vi "SequenceCtrl_HSImaging.vi"(0 "QueuesRef":T2, 1 "MotionStageRefs":refnum<queue>, 2 "AppsRef":refnum<queue>, 3 "subprog_Ref":refnum<vi>, 4 "TotalScan":i32, 5 "SecondaryVI_Ref":refnum<vi>, 7 "Params.":variant, 9 "Laser_Ctrl":bool, 10 "SecendaryParams":variant caption="SecendaryParams (Input)", 11 "error in":errorcluster, 12 "HighSpeed":dbl=5.0, 13 "LowSpeed":dbl=0.1, 14 "Single/MultiRec (T:M)":bool) -> (6 "Interupted":bool, 15 "error out":errorcluster)   [LabVIEW 2014]
uses:
  ControlDef/QueueRefs.ctl
  ControlDef/LaserCtrl_Method.ctl
  ControlDef/States-AToF.ctl
  <instrlib>/GenericDAQ/VI/GenericDAQ_Ctrl_Queue.ctl
  <instrlib>/GenericDAQ/VI/GenericDAQ_State.ctl
  <instrlib>/ESP300/Public/Data/ESP300_State.ctl
  <instrlib>/DG535/Command/DG535_States.ctl
  Hardware/BNC(QuantumComposers)/BNC_States.ctl
  Hardware/FemtoLaser(Legacy)/Laser_Status.ctl
  Hardware/DAQmx(Legacy)/DAQmx_Status.ctl
  ControlDef/Signal.ctl
  ProcessMethods/SignalAverager/ProcessStates.ctl
  Files/WriterState.ctl
  <instrlib>/GenericDAQ/VI/GenericDAQ_Signal.ctl
  Hardware/EPM2000(Legacy)/EPM2K_Status.ctl
  Apps_static/MeanderLoopState.ctl
  SequenceCtrl_State.ctl
  Apps_static/ScanParams_SingleLine.ctl
  <instrlib>/ESP300/Public/Data/ESP30x_Data.ctl
  <vilib>/Utility/error.llb/DialogType.ctl
  <instrlib>/GenericDAQ/VI/InstrParams.vi
  ControlDef/PauseMeander.vi
  <instrlib>/ESP300/ESP300.lvlib
  <instrlib>/DG535/SRS_DG535_Lib.lvlib
  <userlib>/Utility/ErrorLog_lib.lvlib
  <instrlib>/GenericDAQ/GenericDAQ.lvlib
panel:
  out "error out 2":errorcluster
  out "elements":T1[](array[typedef])
  out "timed out?":bool
  out "Core_iter.":i32
  out "Scanned Lines":i32
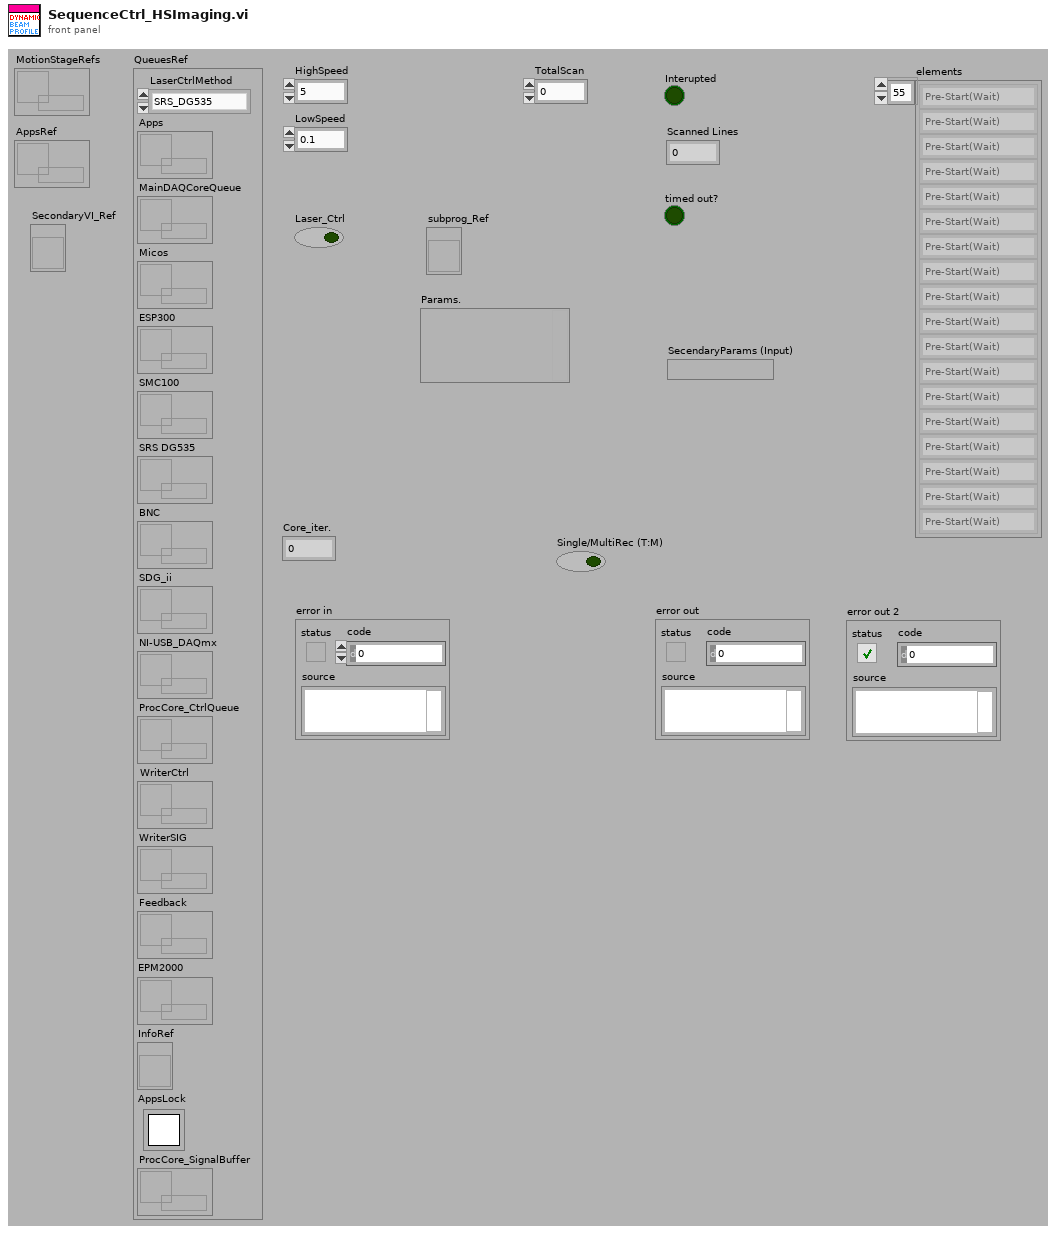
[diagram p1: front panel]
types:
  T1 = typedef "MeanderLoopState.ctl" = enum16{"Pre-Start(Wait)", "Send-loginfo", "SetHighVelocity", "MoveToLineStart", "SetSecondaryParams", "WaitStartReady", "UpdateStartPosition", "StartOfLine", "SetLowVelocity", "MoveToLineEnd", "StartLaser_move", "WaitScanFinish", "StartLaser_still", "KeepStill", "StopLaser", "EndOfLine", "CheckPause", "Exit", "RestoreVelocity", "Pause", "Quit"}
  T2 = typedef "QueueRefs.ctl" = cluster{"LaserCtrlMethod":T3, "Apps":refnum<queue>, "MainDAQCoreQueue":refnum<queue>, "Micos":refnum<queue>, "ESP300":refnum<queue>, "SMC100":refnum<queue>, "SRS DG535":refnum<queue>, "BNC":refnum<queue>, "SDG_ii":refnum<queue>, "NI-USB_DAQmx":refnum<queue>, "ProcCore_CtrlQueue":refnum<queue>, "WriterCtrl":refnum<queue>, "WriterSIG":refnum<queue>, "Feedback":refnum<queue>, "EPM2000":refnum<queue>, "InfoRef":refnum<vi>, "AppsLock":T4, "ProcCore_SignalBuffer":refnum<queue>}
  T3 = typedef "LaserCtrl_Method.ctl" = enum16{"SRS_DG535", "BNC", "SDG_II", "GenericDAQ_Sim"}
  T4 = typedef "Semaphore RefNum" = refnum<k1>
  T5 = typedef "States-AToF.ctl" = enum16{"Initialize", "Idle", "CalcMzArray", "Meander_SGL_MCS", "Meander_MCS", "CleanSurface", "Meander_Npt", "Meander_SGL_Npt", "KnifeEdgeExpt", "KnifeEdgeExpt_Npt", "Imaging_Micos", "Imaging(MultiRec)", "DepthProfiling", "Set_2PulseDelay", "DelayScan", "PeakSearch", "ExportOrigin", "Save Settings", "Load Settings", "Save as Default", "Load Default", "EnergyCalibration", "Quit", "Interrupted_Stop", "Quit_SubProgram", "StepMove_Joystick", "ContMove_Joystick", "Stop_Joystick", "Check_AppsLock", "Return_Status", "DepthProfile_RT", "UpdateInstruStates", "InstruOptimizer_static", "InstruOptimizer_dynamic", "DepthProfiling(3D)"}
  T6 = typedef "ScanParams_SingleLine.ctl" = cluster{"Line Start":dbl[], "Line End":dbl[], "HighSpeed":dbl, "ScanSpeed":dbl, "KeepStill(ms)":u32, "SecendaryParams":variant}
  T7 = typedef "SequenceCtrl_State.ctl" = enum16{"Pre-Start(Wait)", "Send-loginfo", "SetHighVelocity", "MoveToLineStart", "SetSecondaryParams", "WaitStartReady", "UpdateStartPosition", "StartOfLine", "SetLowVelocity", "MoveToLineEnd", "StartLaser_move", "WaitScanFinish", "StartLaser_still", "KeepStill", "StopLaser", "EndOfLine", "CheckPause", "Exit", "RestoreVelocity", "Pause", "Quit"}
  T8 = typedef "ESP300.lvlib/ESP300_State.ctl" = cluster{"State":enum16{"Initialize", "SetDefaultConfig", "Close", "Quit", "Identify", "MoveAbs", "MoveAbs_all", "MoveRel", "MoveRel_all", "STOP", "Origin/Home", "WaitStop", "QueryStatus", "UpdateXPos", "UpdateAll", "SetVelocity", "SetAcceleration", "ClearErr", "LogMessage", "MotorEnable(1)", "EnableAxis", "JoyStick", "GetVelocity", "GetAcceleration", "SendCmd", "SetSoftLimits", "Beep", "_SettingReturn", "SoftReset"}, "Params.":variant}
  T9 = typedef "ESP300.lvlib/ESP30x_Data.ctl" = cluster{"Position":dbl[], "Velocity":dbl[], "Acceleration":dbl[], "Moving":bool, "Simulation":bool, "tickcount_mov":u32, "tickcount_pos":u32, "NumOfAxis":i32, "Initialized":bool, "CommPort":refnum<visa-resource-name>, "Range":dbl[][], "Serial Configuration":cluster{"Baud Rate":u32, "Parity":u16, "Data Bits":u16, "Stop Bits":u16, "Flow Control":u16}, "MotorDisabled":refnum<vi>}
  T10 = typedef "GenericDAQ.lvlib/GenericDAQ_Ctrl_Queue.ctl" = cluster{"GenericDAQ State":T11, "Variant":variant}
  T11 = typedef "GenericDAQ.lvlib/GenericDAQ_State.ctl" = enum16{"Enumerate", "Open", "Close", "CloseAll", "Reset", "Quit", "==Settings==", "SetAcquisition_", "SetChannels_", "SetTrigger_", "SetAnalogTrigDetector_", "SetSegment#_", "SetAll_AcquChTrig_", "fConfigurate", "fStart", "GetStatus", "_WaitForDone/Idle", "_GetData", "GetAcquisition", "GetChannels", "GetTrigger", "GetAll_AcquChTrig", "Abort", "==Messaging==", "_PushDataOut", "GetStat_", "GetConfig_", "==ModeSetup==", "SetSignalBuffer_", "SetMode_", "SetSecondaryDataRef._", "SetDynamicBuffer_", "==AnalogOut==", "GetChannelCount_AO", "fStart_AO", "SetChEnable_AO", "SetConfig_AO", "SetFuncData_AO", "SetOffset_AO_", "SetMasterNode_AO", "SetStates_AO", "SetSymetry_AO", "SetTriggerSource_AO", "==Trigger==", "ManualTrigger", "===Sync===", "LineStart", "LineEnd", "FrameStart", "FrameEnd", "EOL_PassThrough", "SOL_PassThrough"}
  T12 = typedef "Laser_Status.ctl" = cluster{"State":enum16{"Initialize", "Idle/Update", "Configure", "Turn On", "Tun OFF", "Continuous", "Single Shot", "ManualTrigger", "Close", "Quit"}, "Parameter":dbl}
  T13 = typedef "BNC_States.ctl" = cluster{"State":enum16{"Initialize", "Set System", "Set C-Input", "Set C-Mode", "Set C-Output", "Set C-Enable", "Manl_Trig", "Run", "Stop", "Query C Number", "Query Status", "Close", "Quit"}, "Para.":variant}
  T14 = typedef "SRS_DG535_Lib.lvlib/DG535_States.ctl" = cluster{"State":enum16{"Initialize", "Set Trigger", "Set Output", "Set Delay", "Manl_Trig", "Run", "Stop", "Close", "Quit"}, "Para.":variant}
  T15 = enum16{"Pre-Start", "Send-loginfo", "SetHighVelocity", "MoveToLineStart", "WaitStartReady", "UpdateStartPosition", "StartOfLine", "SetLowVelocity", "MoveToLineEnd", "StartLaser", "WaitScanFinish", "StopLaser", "EndOfLine", "CheckPause", "Exit", "RestoreHighVelocity", "Pause"}
  T16 = cluster{"Line Start[0]":dbl, "Line Start[1]":dbl, "Line Start[2]":dbl}
  T17 = cluster{"Line End[0]":dbl, "Line End[1]":dbl, "Line End[2]":dbl}
  T18 = typedef "DialogType.ctl" = u16
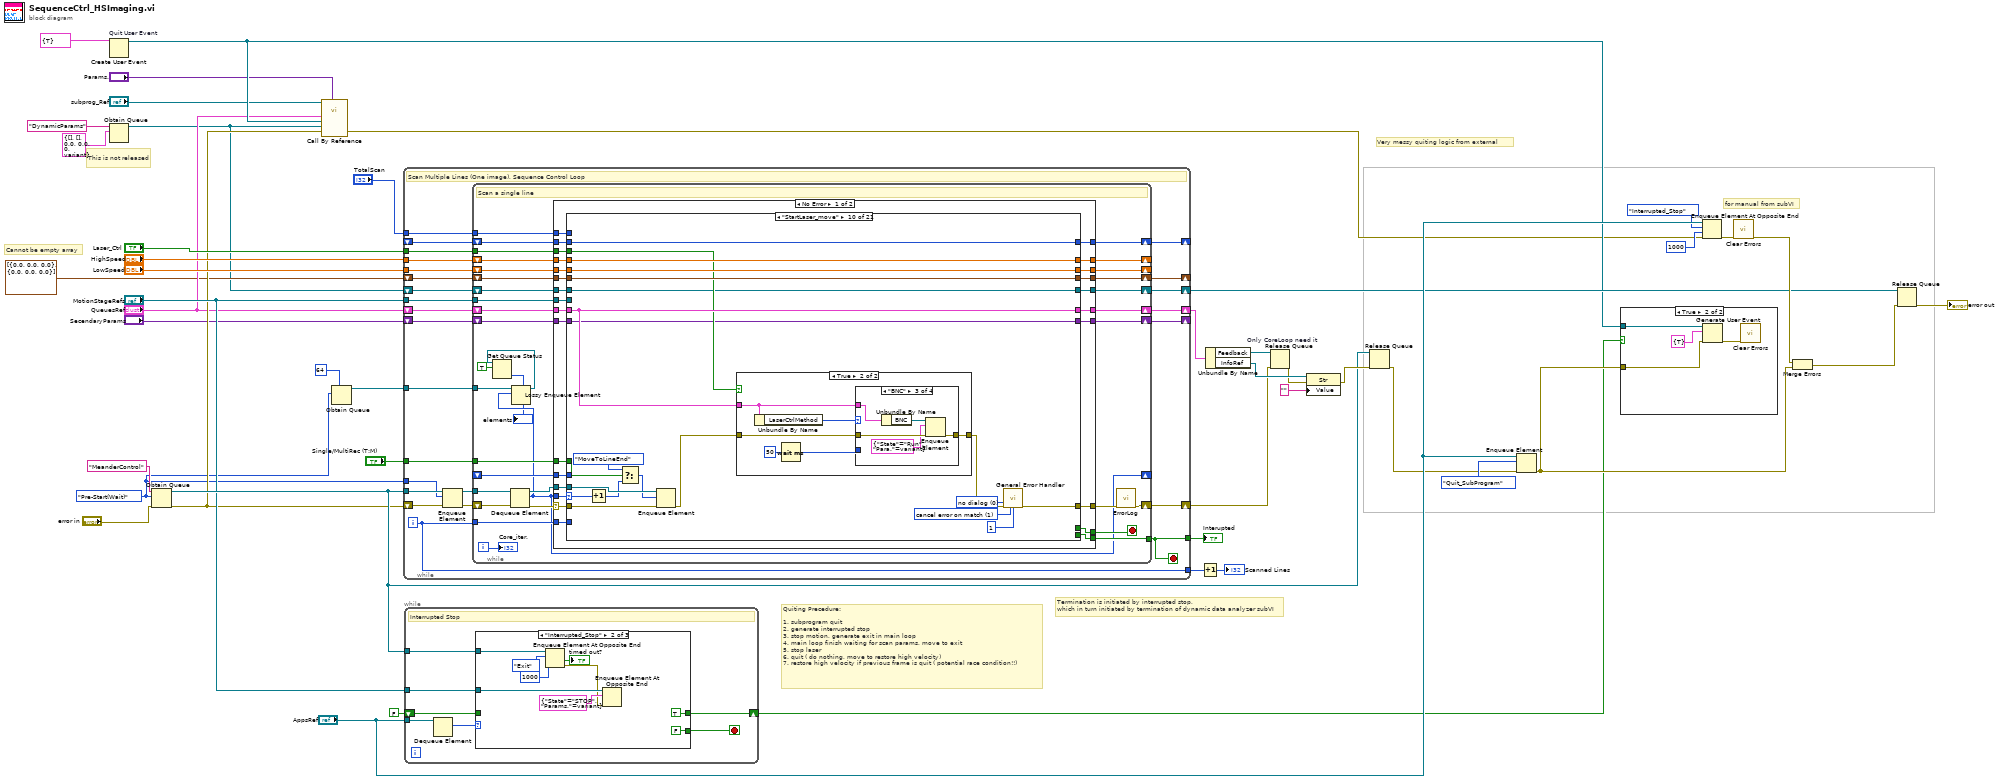
[diagram p0: block diagram]
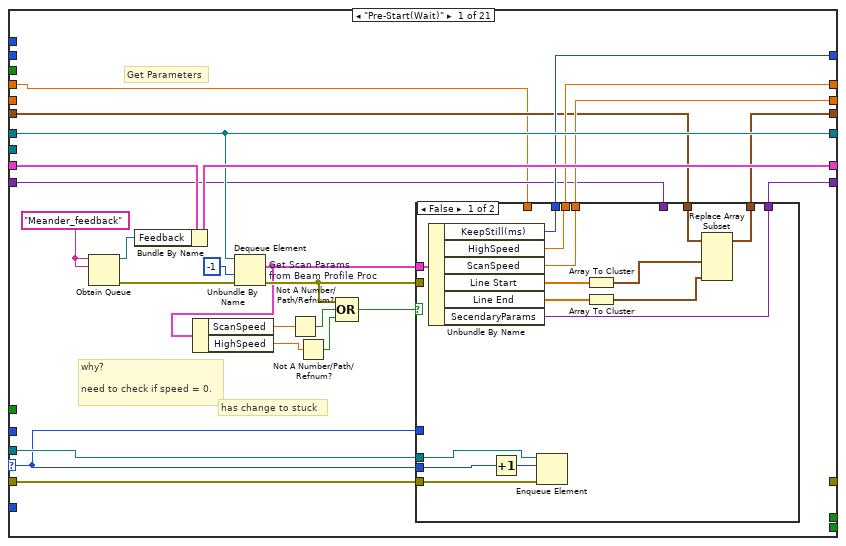
[diagram p2: hidden frame]
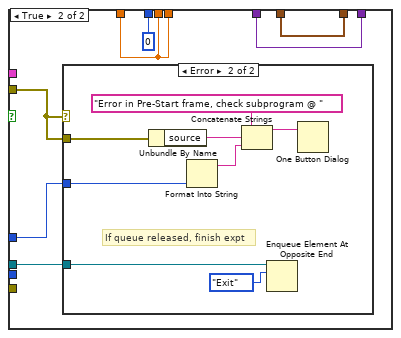
[diagram p3: hidden frame]
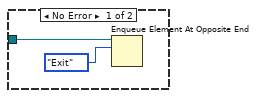
[diagram p4: hidden frame]
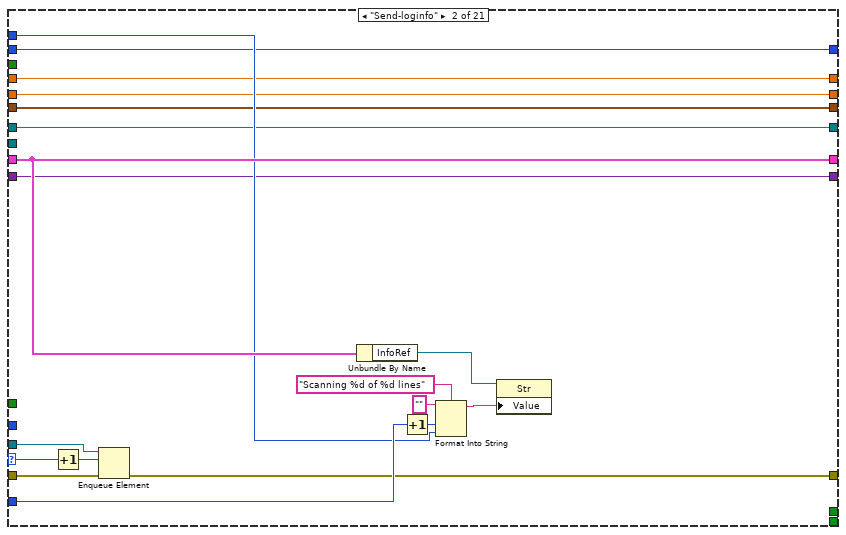
[diagram p5: hidden frame]
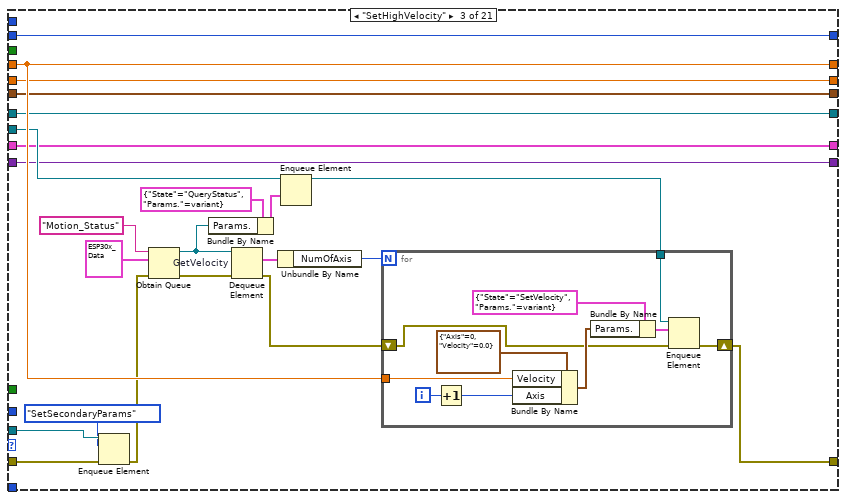
[diagram p6: hidden frame]
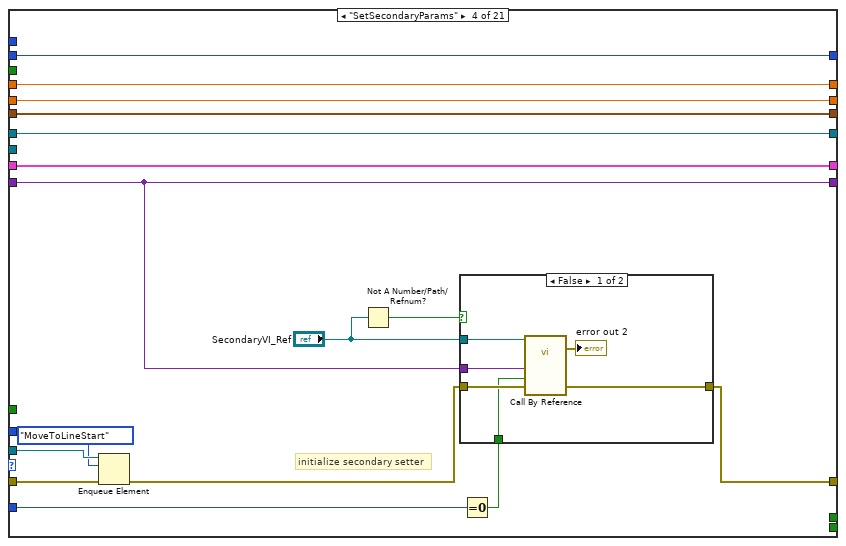
[diagram p7: hidden frame]
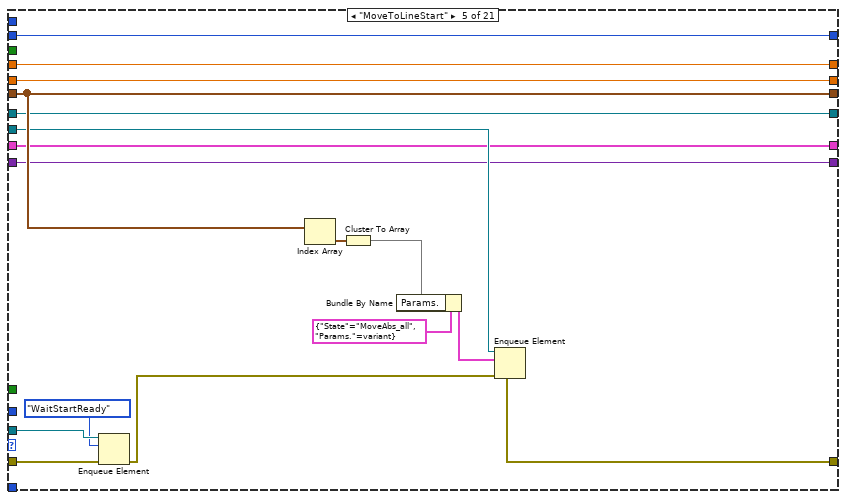
[diagram p9: hidden frame]
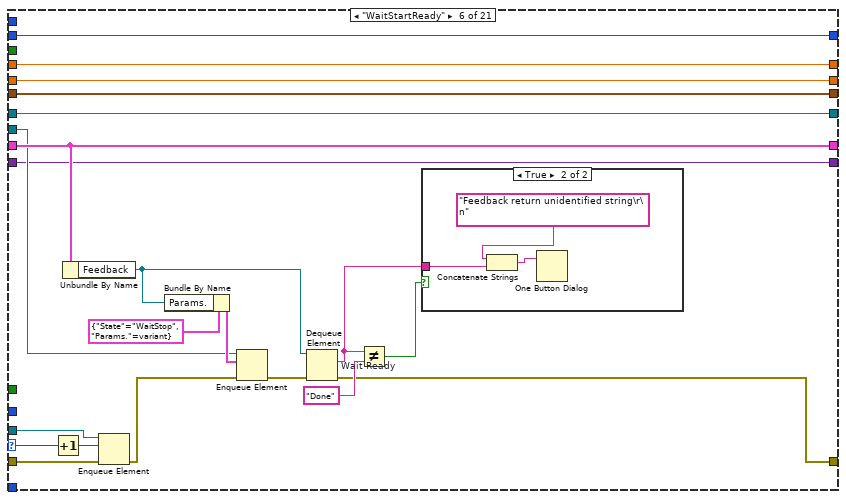
[diagram p10: hidden frame]
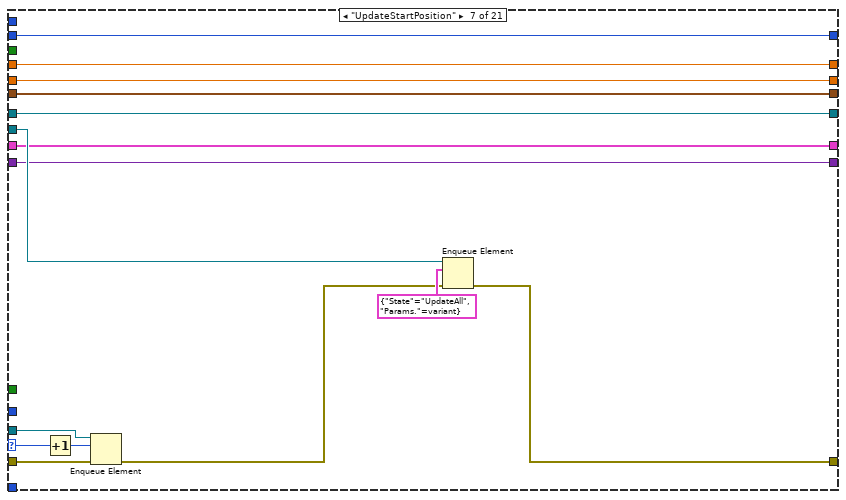
[diagram p12: hidden frame]
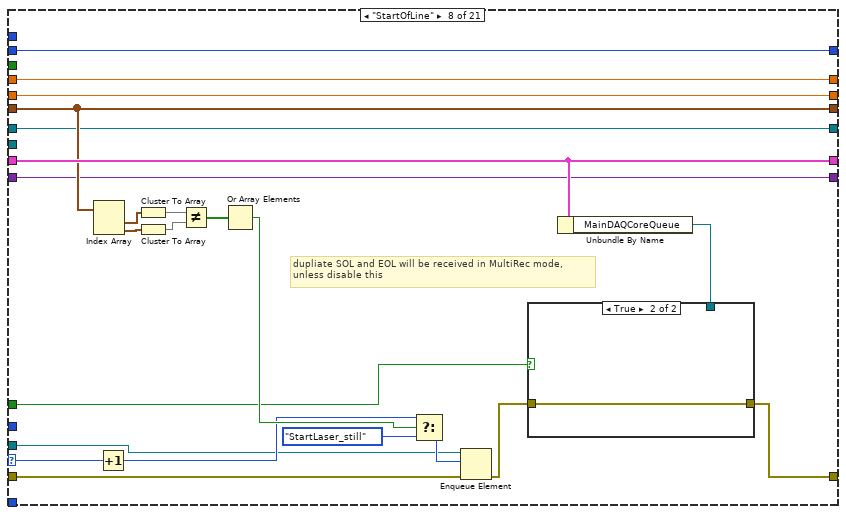
[diagram p13: hidden frame]
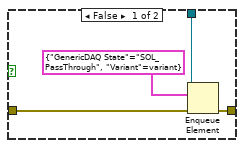
[diagram p14: hidden frame]
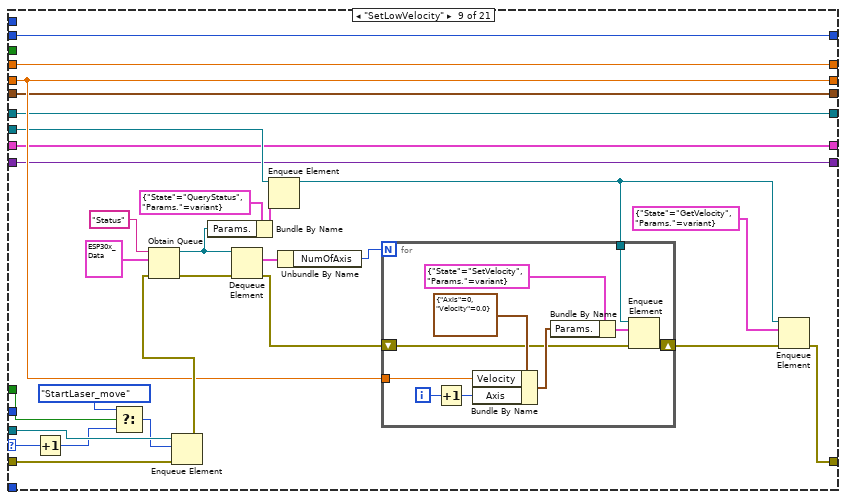
[diagram p15: hidden frame]
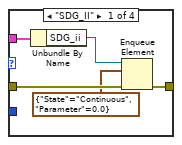
[diagram p17: hidden frame]
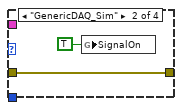
[diagram p18: hidden frame]
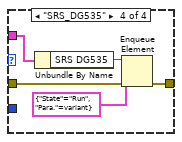
[diagram p19: hidden frame]
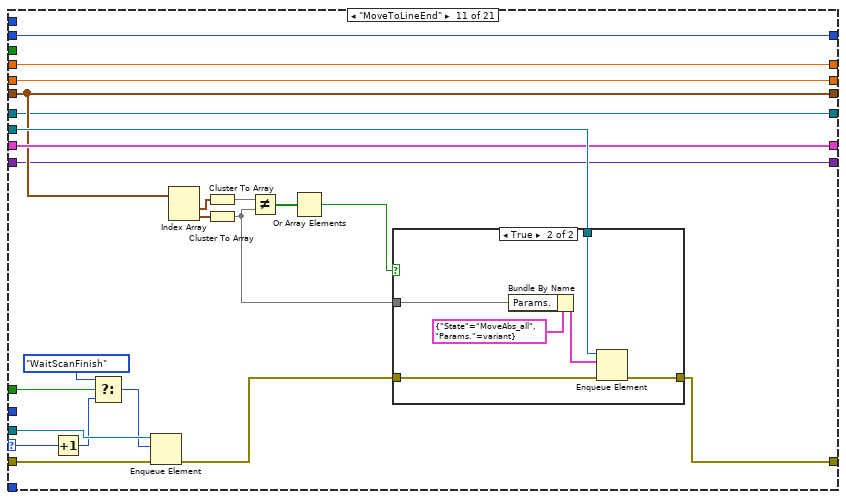
[diagram p20: hidden frame]
diagram:
  w3 = SequenceCtrl_State."Pre-Start(Wait)"
  # "Termination is initiated by interrupted stop, \nwhich in turn initiated by termination of dynamic data analyzer subVI"
  # "Cannot be empty array"
  # "Quiting Precedure:\n\n1. subprogram quit\n2. generate interrupted stop\n3. stop motion, generate exit in main loop\n4. main loop finish waiting for scan params, move to exit \n5. stop laser\n6. quit ( do nothing, move to restore high velocity)\n7. restore high velocity if previous frame is quit ( potential race condition!!)"
  # "Very messy quiting logic from external"
  # "This is not released"
  # "for manual from subVI"
  n1 = Create User Event "Quit User Event"(user event datatype=cluster{"Quit":bool} {"Quit"=TRUE} ("Quit")) -> (user event=w14:refnum<user-event>)  [unwired: 1 in, 1 out]
  n2 = Obtain Queue(name (unnamed)="DynamicParams", element data type=T6 {"Line Start"=[], "Line End"=[], "HighSpeed"=0.0, "ScanSpeed"=0.0, "KeepStill(ms)"=0, "SecendaryParams"=variant}) -> (queue out=w4:refnum<queue>)  [unwired: 3 in, 2 out]
  n3 = Obtain Queue(name (unnamed)="MeanderControl", element data type=w3, error in (no error)="error in") -> (queue out=w27:refnum<queue>, error out=w13:errorcluster)  [unwired: 2 in, 1 out]
  n4 = call-by-ref "?"(reference="subprog_Ref", "Params."="Params.", "error in (no error)"=w13, "Dynamic Params queue"=w4, "Quit_UserEvent"=w14, "ControlQueueRef"="QueuesRef") -> ("error out"=w12:errorcluster)  [unwired: 6 in, 3 out]
  n5 = Obtain Queue(max queue size (-1, unlimited)=64, element data type=w3) -> (queue out=w1:refnum<queue>)  [unwired: 3 in, 2 out]
  n6 = while {
    tunnel: "MotionStageRefs" -> [w71]
    tunnel: w27 -> [w67]
    tunnel: "Laser_Ctrl" -> [w66]
    tunnel: [w65] -> w45
    shift-right: [w64] -> w33
    shift-left: w13 -> [w63]
    tunnel: [w62] -> w42
    tunnel: w3 -> [w60]
    shift-right: [w59] -> w35
    shift-left: "QueuesRef" -> [w70]
    tunnel: "HighSpeed" -> [w68]
    tunnel: "LowSpeed" -> [w69]
    shift-right: [w54] -> w20
    shift-left: w4 -> [w58]
    shift-right: [w53] -> _
    shift-left: _ -> [w57]
    tunnel: "TotalScan" -> [w52]
    shift-right: [w55] -> _
    shift-left: cluster{dbl, dbl, dbl}[] [{0.0, 0.0, 0.0}, {0.0, 0.0, 0.0}] ("start/end points") -> [w56]
    tunnel: "Single/MultiRec (T:M)" -> [w51]
    shift-right: [w49] -> _
    shift-left: "SecendaryParams" -> [w50]
    tunnel: w1 -> [w48]
    i -> [w65]
    stop <- w62 stop-if-true
    # "Scan Multiple Lines (One image), Sequence Control Loop"
    n7 = Enqueue Element(queue=w67, element=w60) -> (queue out=w61:refnum<queue>)  [unwired: 2 in, 2 out]
    n8 = while {
      tunnel: w71 -> [w105]
      tunnel: w61 -> [w101]
      tunnel: w65 -> [w99]
      shift-right: [w80] -> w64
      shift-left: w63 -> [w82]
      tunnel: w66 -> [w96]
      shift-right: [w75] -> _
      shift-left: _ -> [w95]
      tunnel: [w94] -> w62
      tunnel: w52 -> [w93]
      shift-right: [w92] -> w59
      shift-left: w70 -> [w104]
      shift-right: [w90] -> _
      shift-left: w68 -> [w102]
      shift-right: [w91] -> _
      shift-left: w69 -> [w103]
      shift-right: [w86] -> w53
      shift-left: w57 -> [w88]
      shift-right: [w87] -> w55
      shift-left: w56 -> [w85]
      shift-right: [w81] -> w54
      shift-left: w58 -> [w89]
      tunnel: w51 -> [w79]
      tunnel: w48 -> [w76]
      shift-right: [w77] -> w49
      shift-left: w50 -> [w78]
      i -> [w84]
      stop <- w100 stop-if-true
      # "Scan a single line"
      n9 = Dequeue Element(queue=w101, error in (no error)=w82) -> (queue out=w98:refnum<queue>, element=w75:T7, error out=w83:errorcluster)  [unwired: 1 in, 1 out]
      n10 = Lossy Enqueue Element(queue=w76, element=w75) -> (queue out=w74:refnum<queue>)  [unwired: 1 in, 3 out]
      n11 = Get Queue Status(queue=w74, return elements? (F)=TRUE) -> (elements=→"elements":T7[])  [unwired: 1 in, 7 out]
      n12 = case shown="No Error" w83 {
        selector: w83 -> [w110 w753]
        tunnel: w105 -> [w131 _]
        tunnel: w104 -> [w130 w757]
        tunnel: w103 -> [w129 w756]
        tunnel: w102 -> [w128 w755]
        tunnel: [w127 _] -> w100
        tunnel: w99 -> [w126 _]
        tunnel: w98 -> [w125 _]
        tunnel: [w124 _] -> w97
        tunnel: w96 -> [w123 _]
        tunnel: w75 -> [w122 _]
        tunnel: w95 -> [w121 w748]
        tunnel: [w120 _] -> w94
        tunnel: w93 -> [w119 _]
        tunnel: [w118 w757] -> w92
        tunnel: [w117 w756] -> w91
        tunnel: [w116 w755] -> w90
        tunnel: w89 -> [w115 w751]
        tunnel: w88 -> [w114 w754]
        tunnel: [w113 w747] -> w87
        tunnel: [w112 w754] -> w86
        tunnel: w85 -> [w111 w747]
        tunnel: [w109 w751] -> w81
        tunnel: w79 -> [w108 _]
        tunnel: w78 -> [w107 w746]
        tunnel: [w106 w746] -> w77
        frame No Error {
          n13 = case shown="\"StartLaser_move\"" w122 {
            selector: w122 -> [w135 w207 _ _ _ w301 w319 w325 w376 w407 w454 w482 w503 w537 w554 _ _ _ _ _ _]
            tunnel: w131 -> [_ _ w215 _ w271 w287 w314 _ w363 _ w449 w468 _ _ _ _ _ w640 w658 _ w723]
            tunnel: w130 -> [w156 w202 w214 w253 w270 w299 w311 w342 w362 w399 w448 w480 w493 w535 w550 w590 w604 w634 w657 w687 w722]
            tunnel: w129 -> [_ w193 w213 w251 w268 w285 w309 w338 w364 w403 w446 w466 w498 w530 w546 w586 w602 w632 w656 w685 w721]
            tunnel: w128 -> [w134 w194 w228 w252 w269 w286 w310 w339 w360 w404 w447 w467 w499 w531 w547 w587 w603 w633 w670 w686 w735]
            tunnel: [_ _ _ _ _ _ _ _ _ _ _ _ _ _ _ _ TRUE FALSE _ _ w716] -> w127
            tunnel: w126 -> [_ w200 _ w243 _ _ _ _ _ _ _ _ _ _ _ _ _ _ _ _ _]
            tunnel: w125 -> [w137 w199 w230 w256 w280 w298 w317 w326 w375 w406 w453 w479 w501 w534 w552 w592 w607 w625 w651 w691 _]
            tunnel: w110 -> [w136 w198 w229 w255 w279 w297 w316 w327 w374 w405 w452 w478 w500 w533 w551 w591 w608 w641 w652 w694 w717]
            tunnel: [_ w197 w217 w245 w272 w288 w312 w340 w355 w396 w450 w469 w490 w532 w541 w588 w605 _ w660 w693 w725] -> w124
            tunnel: w111 -> [w147 w192 w212 w254 w276 w284 w308 w324 w359 w402 w440 w465 w497 w529 w545 w585 w601 w631 w655 w684 w720]
            tunnel: w123 -> [_ _ _ _ _ _ _ _ _ w398 _ _ w494 _ w549 _ _ _ _ _ _]
            tunnel: w121 -> [_ _ _ _ _ _ _ _ _ _ _ _ _ _ _ _ _ _ _ _ _]
            tunnel: [_ _ _ _ _ _ _ _ _ _ _ _ _ _ _ _ w606 _ _ _ w716] -> w120
            tunnel: w119 -> [_ w195 _ _ _ _ _ _ _ _ _ _ _ _ _ _ _ _ _ _ _]
            tunnel: [w155 w202 w214 w253 w270 w299 w311 w342 w362 w399 w448 w480 w493 w535 w550 w590 w604 w634 w657 w687 w722] -> w118
            tunnel: [w150 w193 w213 w251 w268 w285 w309 w338 w364 w403 w446 w466 w498 w530 w546 w586 w602 w632 w656 w685 w721] -> w117
            tunnel: [w151 w194 w228 w252 w269 w286 w310 w339 w360 w404 w447 w467 w499 w531 w547 w587 w603 w633 w670 w686 w735] -> w116
            tunnel: w115 -> [w152 w190 w210 w249 w266 w282 w306 w322 w353 w392 w437 w463 w488 w527 w540 w583 w599 w626 w653 w682 w718]
            tunnel: w114 -> [_ w191 w211 w250 w267 w283 w307 w337 w358 w401 w445 w464 w495 w528 w544 w584 w600 w630 w654 w683 w719]
            tunnel: [w146 w192 w212 w254 w276 w284 w308 w324 w359 w402 w440 w465 w497 w529 w545 w585 w601 w631 w655 w684 w720] -> w113
            tunnel: [w149 w191 w211 w250 w267 w283 w307 w337 w358 w401 w445 w464 w495 w528 w544 w584 w600 w630 w654 w683 w719] -> w112
            tunnel: [w152 w190 w210 w249 w266 w282 w306 w322 w353 w392 w437 w463 w488 w527 w540 w583 w599 w626 w653 w682 w718] -> w109
            tunnel: w108 -> [_ _ _ _ _ _ _ w320 w349 w388 w433 _ _ _ _ w579 _ _ _ _ _]
            tunnel: w107 -> [w138 w189 w209 w244 w265 w281 w305 w321 w348 w387 w432 w462 w487 w526 w539 w580 w598 w624 w648 w681 w715]
            tunnel: [w139 w189 w209 w244 w265 w281 w305 w321 w348 w387 w432 w462 w487 w526 w539 w580 w598 w624 w648 w681 w715] -> w106
            frame "Pre-Start(Wait)" {
              w153 = "Meander_feedback" ("name (unnamed)")
              # "Get Parameters"
              # "why?\n\nneed to check if speed = 0."
              # "has change to stuck"
              n14 = Obtain Queue(name (unnamed)=w153, element data type=w153) -> (queue out=w154:refnum<queue>, error out=w148:errorcluster)  [unwired: 3 in, 1 out]
              n15 = Bundle By Name(cluster=w156, "Feedback"=w154) -> (w155:T2)
              n16 = Dequeue Element "Get Scan Params\nfrom Beam Profile Proc"(queue=w152, timeout in ms (-1)=-1, error in (no error)=w148) -> (element=w142:T6, error out=w143:errorcluster)  [unwired: 2 out]
              n17 = Unbundle By Name(w142) -> ("ScanSpeed"=w141:dbl, "HighSpeed"=w133:dbl)
              n18 = Not A Number/Path/Refnum?(number/path/refnum=w141) -> (NaN/Path/Refnum?=w140:bool)
              n19 = Not A Number/Path/Refnum?(number/path/refnum=w133) -> (NaN/Path/Refnum?=w132:bool)
              n20 = Compound Arithmetic op=OR(w143, w140, w132) -> (w144:bool)
              n21 = case shown="False" w144 {
                tunnel: w142 -> [w171 _]
                tunnel: [w170 w172] -> w151
                tunnel: [w169 w172] -> w150
                tunnel: [w168 u32 0 ("KeepStill(ms)")] -> w149
                tunnel: w147 -> [w165 w175]
                tunnel: [w164 w175] -> w146
                tunnel: w143 -> [_ w178]
                tunnel: w135 -> [_ w177]
                tunnel: w137 -> [w160 w174]
                tunnel: [w157 w173] -> w139
                tunnel: w138 -> [_ w173]
                tunnel: w136 -> [w159 _]
                tunnel: w135 -> [w158 _]
                tunnel: w134 -> [_ w172]
                frame False {
                  n22 = Unbundle By Name(w171) -> ("KeepStill(ms)"=w168:u32, "HighSpeed"=w170:dbl, "ScanSpeed"=w169:dbl, "Line Start"=w167:dbl[], "Line End"=w166:dbl[], "SecendaryParams"=w157:variant)
                  n23 = Increment(x=w158) -> (x+1=w161:T7)
                  n24 = Enqueue Element(queue=w160, element=w161, error in (no error)=w159) -> ()  [unwired: 1 in, 3 out]
                  n25 = Array To Cluster(array=w167) -> (cluster=w163:T16)
                  n26 = Array To Cluster(array=w166) -> (cluster=w162:T17)
                  n27 = Replace Array Subset(array=w165, new element #1=w163, new element #2=w162) -> (w164:cluster{dbl, dbl, dbl}[])  [unwired: 2 in]
                }
                frame True {
                  n28 = case shown="Error" w178 {
                    tunnel: w178 -> [_ w185]
                    tunnel: w177 -> [_ w184]
                    tunnel: w174 -> [w180 w182]
                    frame No Error {
                      n29 = Enqueue Element At Opposite End(queue=w180, element=SequenceCtrl_State."Exit") -> ()  [unwired: 2 in, 3 out]
                    }
                    frame Error {
                      # "If queue released, finish expt"
                      n30 = Unbundle By Name(w185) -> ("source"=w186:string)
                      n31 = Format Into String(w184) -> (resulting string=w183:string)  [unwired: 3 in, 1 out]
                      n32 = Concatenate Strings("Error in Pre-Start frame, check subprogram @ " ("message"), w186, w183) -> (w188:string)
                      n33 = Enqueue Element At Opposite End(queue=w182, element=SequenceCtrl_State."Exit") -> ()  [unwired: 2 in, 3 out]
                      n34 = One Button Dialog(message=w188) -> ()  [unwired: 1 in, 1 out]
                    }
                  }
                }
              }
            }
            frame "Send-loginfo" {
              n35 = Increment(x=w207) -> (x+1=w206:T7)
              n36 = Enqueue Element(queue=w199, element=w206, error in (no error)=w198) -> (error out=w197:errorcluster)  [unwired: 1 in, 2 out]
              n37 = Unbundle By Name(w202) -> ("InfoRef"=w201:refnum<vi>)
              n38 = Increment(x=w200) -> (x+1=w204:i32)
              n39 = Format Into String(format string="Scanning %d of %d lines", initial string="", w204, w195) -> (resulting string=w205:string)  [unwired: 1 in, 1 out]
              n40 = property class="Str"(reference=w201, "Value"=w205) -> ()  [unwired: 1 in, 2 out]
            }
            frame "SetHighVelocity" {
              n41 = Enqueue Element(queue=w230, element=SequenceCtrl_State."SetSecondaryParams", error in (no error)=w229) -> (error out=w218:errorcluster)  [unwired: 1 in, 2 out]
              n42 = Obtain Queue(name (unnamed)="Motion_Status", element data type=T9 {"Position"=[], "Velocity"=[], "Acceleration"=[], "Moving"=FALSE, "Simulation"=FALSE, "tickcount_mov"=0, "tickcount_pos"=0, "NumOfAxis"=0, "Initialized"=FALSE, "CommPort"="", "Range"=[], "Serial Configuration"={"Baud Rate"=0, "Parity"=0, "Data Bits"=0, "Stop Bits"=0, "Flow Control"=0}, "MotorDisabled"=refnum}, error in (no error)=w218) -> (queue out=w223:refnum<queue>, error out=w222:errorcluster)  [unwired: 2 in, 1 out]
              n43 = Bundle By Name(cluster=T8 {"State"=enum."QueryStatus", "Params."=variant} ("element"), "Params."=w223) -> (w224:T8)
              n44 = Dequeue Element "GetVelocity"(queue=w223, error in (no error)=w222) -> (element=w221:T9, error out=w219:errorcluster)  [unwired: 1 in, 2 out]
              n45 = Unbundle By Name(w221) -> ("NumOfAxis"=w220:i32)
              n46 = Enqueue Element(queue=w215, element=w224) -> (queue out=w227:refnum<queue>)  [unwired: 2 in, 2 out]
              n47 = for {
                N: w220 -> [_]
                tunnel: w227 -> [w234]
                tunnel: w228 -> [w233]
                shift-right: [w231] -> w217
                shift-left: w219 -> [w232]
                i -> [w240]
                n48 = Increment(x=w240) -> (x+1=w238:i32)
                n49 = Bundle By Name(cluster=cluster{"Axis":i32, "Velocity":dbl} {"Axis"=0, "Velocity"=0.0}, "Velocity"=w233, "Axis"=w238) -> (w235:cluster{"Axis":i32, "Velocity":dbl})
                n50 = Bundle By Name(cluster=T8 {"State"=enum."SetVelocity", "Params."=variant} ("element"), "Params."=w235) -> (w237:T8)
                n51 = Enqueue Element(queue=w234, element=w237, error in (no error)=w232) -> (error out=w231:errorcluster)  [unwired: 1 in, 2 out]
              }
            }
            frame "SetSecondaryParams" {
              # "initialize secondary setter"
              n52 = Enqueue Element(queue=w256, element=SequenceCtrl_State."MoveToLineStart", error in (no error)=w255) -> (error out=w246:errorcluster)  [unwired: 1 in, 2 out]
              n53 = Not A Number/Path/Refnum?(number/path/refnum="SecondaryVI_Ref") -> (NaN/Path/Refnum?=w248:bool)
              n54 = Equal To 0?(x=w243) -> (x = 0?=w242:bool)
              n55 = case shown="False" w248 {
                tunnel: w246 -> [w262 w263]
                tunnel: [w260 w263] -> w245
                tunnel: "SecondaryVI_Ref" -> [w261 _]
                tunnel: w244 -> [w259 _]
                tunnel: w242 -> [w258 _]
                frame False {
                  n56 = call-by-ref "?"(reference=w261, "error in"=w262, "WaitForReady"=w258, "InputParams."=w259) -> (error out=→"error out 2":errorcluster, 0:"error out"=w260:errorcluster)  [unwired: 8 in, 2 out]
                }
                frame True {
                }
              }
            }
            frame "MoveToLineStart" {
              n57 = Enqueue Element(queue=w280, element=SequenceCtrl_State."WaitStartReady", error in (no error)=w279) -> (error out=w273:errorcluster)  [unwired: 1 in, 2 out]
              n58 = Index Array(array=w276) -> (element=w275:cluster{dbl, dbl, dbl})  [unwired: 1 in]
              n59 = Cluster To Array(cluster=w275) -> (array=w274:dbl[])
              n60 = Bundle By Name(cluster=T8 {"State"=enum."MoveAbs_all", "Params."=variant} ("element"), "Params."=w274) -> (w277:T8)
              n61 = Enqueue Element(queue=w271, element=w277, error in (no error)=w273) -> (error out=w272:errorcluster)  [unwired: 1 in, 2 out]
            }
            frame "WaitStartReady" {
              n62 = Increment(x=w301) -> (x+1=w300:T7)
              n63 = Unbundle By Name(w299) -> ("Feedback"=w292:refnum<queue>)
              n64 = Enqueue Element(queue=w298, element=w300, error in (no error)=w297) -> (error out=w294:errorcluster)  [unwired: 1 in, 2 out]
              n65 = Bundle By Name(cluster=T8 {"State"=enum."WaitStop", "Params."=variant} ("element"), "Params."=w292) -> (w295:T8)
              n66 = Enqueue Element(queue=w287, element=w295, error in (no error)=w294) -> (error out=w293:errorcluster)  [unwired: 1 in, 2 out]
              n67 = Dequeue Element "Wait Ready"(queue=w292, error in (no error)=w293) -> (element=w289:string, error out=w288:errorcluster)  [unwired: 1 in, 2 out]
              n68 = Not Equal?(x=w289, y="Done" ("element")) -> (x != y?=w290:bool)
              n69 = case shown="True" w290 {
                tunnel: w289 -> [_ w303]
                frame False {
                }
                frame True {
                  n70 = Concatenate Strings("Feedback return unidentified string\r\n" ("message"), w303) -> (w304:string)
                  n71 = One Button Dialog(message=w304) -> ()  [unwired: 1 in, 1 out]
                }
              }
            }
            frame "UpdateStartPosition" {
              n72 = Increment(x=w319) -> (x+1=w318:T7)
              n73 = Enqueue Element(queue=w317, element=w318, error in (no error)=w316) -> (error out=w313:errorcluster)  [unwired: 1 in, 2 out]
              n74 = Enqueue Element(queue=w314, element=T8 {"State"=enum."UpdateAll", "Params."=variant}, error in (no error)=w313) -> (error out=w312:errorcluster)  [unwired: 1 in, 2 out]
            }
            frame "StartOfLine" {
              # "dupliate SOL and EOL will be received in MultiRec mode, \nunless disable this"
              n75 = Index Array(array=w324) -> (element #1=w330:cluster{dbl, dbl, dbl}, element #2=w329:cluster{dbl, dbl, dbl})  [unwired: 2 in]
              n76 = Increment(x=w325) -> (x+1=w334:T7)
              n77 = Cluster To Array(cluster=w330) -> (array=w331:dbl[])
              n78 = Cluster To Array(cluster=w329) -> (array=w332:dbl[])
              n79 = Not Equal?(x=w331, y=w332) -> (x != y?=w333:bool[])
              n80 = Or Array Elements(Boolean array=w333) -> (logical OR=w336:bool)
              n81 = Select(t=w334, s=w336, f=SequenceCtrl_State."StartLaser_still") -> (s? t:f=w328:T7)
              n82 = Enqueue Element(queue=w326, element=w328, error in (no error)=w327) -> (error out=w323:errorcluster)  [unwired: 1 in, 2 out]
              n83 = Unbundle By Name(w342) -> ("MainDAQCoreQueue"=w341:refnum<queue>)
              n84 = case shown="True" w320 {
                tunnel: w341 -> [w346 _]
                tunnel: [w345 w347] -> w340
                tunnel: w323 -> [w344 w347]
                frame False {
                  n85 = Enqueue Element(queue=w346, element=T10 {"GenericDAQ State"=enum."SOL_PassThrough", "Variant"=variant}, error in (no error)=w344) -> (error out=w345:errorcluster)  [unwired: 1 in, 2 out]
                }
                frame True {
                }
              }
            }
            frame "SetLowVelocity" {
              n86 = Increment(x=w376) -> (x+1=w351:T7)
              n87 = Select(t=SequenceCtrl_State."StartLaser_move" ("f"), s=w349, f=w351) -> (s? t:f=w352:T7)
              n88 = Enqueue Element(queue=w375, element=w352, error in (no error)=w374) -> (error out=w365:errorcluster)  [unwired: 1 in, 2 out]
              n89 = Obtain Queue(name (unnamed)="Status", element data type=T9 {"Position"=[], "Velocity"=[], "Acceleration"=[], "Moving"=FALSE, "Simulation"=FALSE, "tickcount_mov"=0, "tickcount_pos"=0, "NumOfAxis"=0, "Initialized"=FALSE, "CommPort"="", "Range"=[], "Serial Configuration"={"Baud Rate"=0, "Parity"=0, "Data Bits"=0, "Stop Bits"=0, "Flow Control"=0}, "MotorDisabled"=refnum}, error in (no error)=w365) -> (queue out=w370:refnum<queue>, error out=w369:errorcluster)  [unwired: 2 in, 1 out]
              n90 = Bundle By Name(cluster=T8 {"State"=enum."QueryStatus", "Params."=variant} ("element"), "Params."=w370) -> (w371:T8)
              n91 = Dequeue Element(queue=w370, error in (no error)=w369) -> (element=w368:T9, error out=w366:errorcluster)  [unwired: 1 in, 2 out]
              n92 = Enqueue Element(queue=w363, element=w371) -> (queue out=w354:refnum<queue>)  [unwired: 2 in, 2 out]
              n93 = Unbundle By Name(w368) -> ("NumOfAxis"=w367:i32)
              n94 = for {
                N: w367 -> [_]
                tunnel: w354 -> [w380]
                tunnel: w364 -> [w379]
                shift-right: [w377] -> w356
                shift-left: w366 -> [w378]
                i -> [w386]
                n95 = Increment(x=w386) -> (x+1=w384:i32)
                n96 = Bundle By Name(cluster=cluster{"Axis":i32, "Velocity":dbl} {"Axis"=0, "Velocity"=0.0}, "Velocity"=w379, "Axis"=w384) -> (w381:cluster{"Axis":i32, "Velocity":dbl})
                n97 = Bundle By Name(cluster=T8 {"State"=enum."SetVelocity", "Params."=variant} ("element"), "Params."=w381) -> (w383:T8)
                n98 = Enqueue Element(queue=w380, element=w383, error in (no error)=w378) -> (error out=w377:errorcluster)  [unwired: 1 in, 2 out]
              }
              n99 = Enqueue Element(queue=w354, element=T8 {"State"=enum."GetVelocity", "Params."=variant}, error in (no error)=w356) -> (error out=w355:errorcluster)  [unwired: 1 in, 2 out]
            }
            frame "StartLaser_move" {
              w393 = T18 0 items=["no dialog", "OK message", "continue or stop message", "OK message + warnings", "continue/stop + warnings"] ("type of dialog (OK msg:1)")
              w395 = 1 items=["no exception", "cancel error on match", "set error on match"] ("[exception action] (none:0)")
              n100 = Increment(x=w407) -> (x+1=w390:T7)
              n101 = Select(t=SequenceCtrl_State."MoveToLineEnd" ("f"), s=w388, f=w390) -> (s? t:f=w389:T7)
              n102 = Enqueue Element(queue=w406, element=w389, error in (no error)=w405) -> (error out=w400:errorcluster)  [unwired: 1 in, 2 out]
              n103 = case shown="True" w398 {
                tunnel: [w408 w414] -> w397
                tunnel: w400 -> [w408 w413]
                tunnel: w399 -> [_ w412]
                frame False {
                }
                frame True {
                  n104 = Unbundle By Name(w412) -> ("LaserCtrlMethod"=w411:T3)
                  n105 = Wait (ms)(milliseconds to wait=u32 50) -> (millisecond timer value=w410:u32)
                  n106 = case shown="\"BNC\"" w411 {
                    tunnel: [w419 w420 w426 w431] -> w414
                    tunnel: w413 -> [w418 w420 w425 w430]
                    tunnel: w412 -> [w416 _ w424 w429]
                    tunnel: w410 -> [_ _ _ _]
                    frame "SDG_II" {
                      n107 = Unbundle By Name(w416) -> ("SDG_ii"=w415:refnum<queue>)
                      n108 = Enqueue Element(queue=w415, element=T12 {"State"=enum."Continuous", "Parameter"=0.0}, error in (no error)=w418) -> (error out=w419:errorcluster)  [unwired: 1 in, 2 out]
                    }
                    frame "GenericDAQ_Sim" {
                      n109 = global write "InstrParams.vi" "SignalOn"(TRUE ("SignalOn")) -> ()
                    }
                    frame "BNC" {
                      n110 = Unbundle By Name(w424) -> ("BNC"=w423:refnum<queue>)
                      n111 = Enqueue Element(queue=w423, element=T13 {"State"=enum."Run", "Para."=variant}, error in (no error)=w425) -> (error out=w426:errorcluster)  [unwired: 1 in, 2 out]
                    }
                    frame "SRS_DG535" {
                      n112 = Unbundle By Name(w429) -> ("SRS DG535"=w428:refnum<queue>)
                      n113 = Enqueue Element(queue=w428, element=T14 {"State"=enum."Run", "Para."=variant}, error in (no error)=w430) -> (error out=w431:errorcluster)  [unwired: 1 in, 2 out]
                    }
                  }
                }
              }
              n114 = call <vilib>:"General Error Handler.vi"("type of dialog (OK msg:1)"=w393, "error in (no error)"=w397, "[exception action] (none:0)"=w395, "[exception code]"=1) -> ("error out"=w396:errorcluster)  [unwired: 7 in, 4 out]
            }
            frame "MoveToLineEnd" {
              n115 = Increment(x=w454) -> (x+1=w434:T7)
              n116 = Select(t=SequenceCtrl_State."WaitScanFinish" ("f"), s=w433, f=w434) -> (s? t:f=w435:T7)
              n117 = Enqueue Element(queue=w453, element=w435, error in (no error)=w452) -> (error out=w451:errorcluster)  [unwired: 1 in, 2 out]
              n118 = Index Array(array=w440) -> (element #1=w442:cluster{dbl, dbl, dbl}, element #2=w441:cluster{dbl, dbl, dbl})  [unwired: 2 in]
              n119 = Cluster To Array(cluster=w442) -> (array=w443:dbl[])
              n120 = Cluster To Array(cluster=w441) -> (array=w439:dbl[])
              n121 = Not Equal?(x=w443, y=w439) -> (x != y?=w444:bool[])
              n122 = Or Array Elements(Boolean array=w444) -> (logical OR=w438:bool)
              n123 = case shown="True" w438 {
                tunnel: w451 -> [w455 w459]
                tunnel: [w455 w458] -> w450
                tunnel: w449 -> [_ w457]
                tunnel: w439 -> [_ w456]
                frame False {
                }
                frame True {
                  n124 = Bundle By Name(cluster=T8 {"State"=enum."MoveAbs_all", "Params."=variant} ("element"), "Params."=w456) -> (w460:T8)
                  n125 = Enqueue Element(queue=w457, element=w460, error in (no error)=w459) -> (error out=w458:errorcluster)  [unwired: 1 in, 2 out]
                }
              }
            }
            frame "WaitScanFinish" {
              n126 = Increment(x=w482) -> (x+1=w481:T7)
              n127 = Unbundle By Name(w480) -> ("Feedback"=w473:refnum<queue>)
              n128 = Enqueue Element(queue=w479, element=w481, error in (no error)=w478) -> (error out=w475:errorcluster)  [unwired: 1 in, 2 out]
              n129 = Bundle By Name(cluster=T8 {"State"=enum."WaitStop", "Params."=variant} ("element"), "Params."=w473) -> (w476:T8)
              n130 = Enqueue Element(queue=w468, element=w476, error in (no error)=w475) -> (error out=w474:errorcluster)  [unwired: 1 in, 2 out]
              n131 = Dequeue Element(queue=w473, error in (no error)=w474) -> (element=w470:string, error out=w469:errorcluster)  [unwired: 1 in, 2 out]
              n132 = Not Equal?(x=w470, y="Done" ("element")) -> (x != y?=w471:bool)
              n133 = case shown="True" w471 {
                tunnel: w470 -> [_ w483]
                frame False {
                }
                frame True {
                  n134 = Concatenate Strings("Feedback return unidentified string\r\n" ("message"), w483) -> (w484:string)
                  n135 = One Button Dialog(message=w484) -> ()  [unwired: 1 in, 1 out]
                }
              }
            }
            frame "StartLaser_still" {
              n136 = Increment(x=w503) -> (x+1=w502:T7)
              n137 = Enqueue Element(queue=w501, element=w502, error in (no error)=w500) -> (error out=w491:errorcluster)  [unwired: 1 in, 2 out]
              n138 = Not Equal To 0?(x=w495) -> (x != 0?=w496:bool)
              n139 = And(x=w496, y=w494) -> (x .and. y?=w492:bool)
              n140 = case shown="True" w492 {
                tunnel: [w504 w508] -> w489
                tunnel: w491 -> [w504 w507]
                tunnel: w493 -> [_ w506]
                frame False {
                }
                frame True {
                  n141 = Unbundle By Name(w506) -> ("LaserCtrlMethod"=w505:T3)
                  n142 = case shown="\"BNC\"" w505 {
                    tunnel: [w513 w518 w519 w525] -> w508
                    tunnel: w507 -> [w512 w517 w519 w524]
                    tunnel: w506 -> [w510 w516 _ w523]
                    frame "SDG_II" {
                      n143 = Unbundle By Name(w510) -> ("SDG_ii"=w509:refnum<queue>)
                      n144 = Enqueue Element(queue=w509, element=T12 {"State"=enum."Continuous", "Parameter"=0.0}, error in (no error)=w512) -> (error out=w513:errorcluster)  [unwired: 1 in, 2 out]
                    }
                    frame "BNC" {
                      n145 = Unbundle By Name(w516) -> ("BNC"=w515:refnum<queue>)
                      n146 = Enqueue Element(queue=w515, element=T13 {"State"=enum."Run", "Para."=variant}, error in (no error)=w517) -> (error out=w518:errorcluster)  [unwired: 1 in, 2 out]
                    }
                    frame "GenericDAQ_Sim" {
                      n147 = global write "InstrParams.vi" "SignalOn"(TRUE ("SignalOn")) -> ()
                    }
                    frame "SRS_DG535" {
                      n148 = Unbundle By Name(w523) -> ("SRS DG535"=w522:refnum<queue>)
                      n149 = Enqueue Element(queue=w522, element=T14 {"State"=enum."Run", "Para."=variant}, error in (no error)=w524) -> (error out=w525:errorcluster)  [unwired: 1 in, 2 out]
                    }
                  }
                }
              }
              n150 = call <vilib>:"Clear Errors.vi"("error in (no error)"=w489, "specific error code to clear (0: all)"=1 ("[exception code]")) -> ("error out"=w490:errorcluster)  [unwired: 4 in, 1 out]
            }
            frame "KeepStill" {
              n151 = Increment(x=w537) -> (x+1=w536:T7)
              n152 = Enqueue Element(queue=w534, element=w536, error in (no error)=w533) -> (error out=w532:errorcluster)  [unwired: 1 in, 2 out]
              n153 = case shown="Default" w528 {
                selector: w528 -> [_ w538]
                frame 0 {
                }
                frame Default {
                  n154 = Wait (ms)(milliseconds to wait=w538) -> ()  [unwired: 1 out]
                }
              }
            }
            frame "StopLaser" {
              # "wait for multirec finish then stoplaser"
              n155 = Increment(x=w554) -> (x+1=w553:T7)
              n156 = Enqueue Element(queue=w552, element=w553, error in (no error)=w551) -> (error out=w548:errorcluster)  [unwired: 1 in, 2 out]
              n157 = case shown="True" w549 {
                tunnel: [w555 w557] -> w542
                tunnel: w548 -> [w555 w560]
                tunnel: w550 -> [_ w559]
                frame False {
                }
                frame True {
                  n158 = Unbundle By Name(w559) -> ("LaserCtrlMethod"=w558:T3)
                  n159 = case shown="\"GenericDAQ_Sim\"" w558 {
                    tunnel: [w566 w571 w576 w577] -> w561
                    tunnel: w560 -> [w565 w570 w575 w577]
                    tunnel: w559 -> [w563 w569 w574 _]
                    frame "SDG_II" {
                      n160 = Unbundle By Name(w563) -> ("SDG_ii"=w562:refnum<queue>)
                      n161 = Enqueue Element(queue=w562, element=T12 {"State"=enum."Single Shot", "Parameter"=0.0}, error in (no error)=w565) -> (error out=w566:errorcluster)  [unwired: 1 in, 2 out]
                    }
                    frame "BNC" {
                      n162 = Unbundle By Name(w569) -> ("BNC"=w568:refnum<queue>)
                      n163 = Enqueue Element(queue=w568, element=T13 {"State"=enum."Stop", "Para."=variant}, error in (no error)=w570) -> (error out=w571:errorcluster)  [unwired: 1 in, 2 out]
                    }
                    frame "SRS_DG535" {
                      n164 = Unbundle By Name(w574) -> ("SRS DG535"=w573:refnum<queue>)
                      n165 = Enqueue Element(queue=w573, element=T14 {"State"=enum."Stop", "Para."=variant}, error in (no error)=w575) -> (error out=w576:errorcluster)  [unwired: 1 in, 2 out]
                    }
                    frame "GenericDAQ_Sim" {
                      n166 = global write "InstrParams.vi" "SignalOn"(FALSE ("SignalOn")) -> ()
                    }
                  }
                  n167 = call <userlib>:"Wait (ms)__ogtk.vi"("error in (no error)"=w561, "milliseconds to wait"=u32 50) -> ("error out"=w557:errorcluster)  [unwired: 8 in, 1 out]
                }
              }
              n168 = call <vilib>:"Clear Errors.vi"("error in (no error)"=w542, "specific error code to clear (0: all)"=1 ("[exception code]")) -> ("error out"=w541:errorcluster)  [unwired: 4 in, 1 out]
            }
            frame "EndOfLine" {
              # "Race conditin :\n\nEOL should be sent to Gage,\n\nbefore sent EOL, Gage Buffer needs to be emptied"
              n169 = Enqueue Element(queue=w592, element=SequenceCtrl_State."RestoreVelocity", error in (no error)=w591) -> (error out=w589:errorcluster)  [unwired: 1 in, 2 out]
              n170 = Unbundle By Name(w590) -> ("MainDAQCoreQueue"=w581:refnum<queue>)
              n171 = case shown="True" w579 {
                tunnel: w589 -> [w596 w597]
                tunnel: [w595 w597] -> w588
                tunnel: w581 -> [w594 _]
                frame False {
                  n172 = Enqueue Element(queue=w594, element=T10 {"GenericDAQ State"=enum."EOL_PassThrough", "Variant"=variant}, error in (no error)=w596) -> (error out=w595:errorcluster)  [unwired: 1 in, 2 out]
                }
                frame True {
                }
              }
            }
            frame "CheckPause" {
              # "Finish single Cycle"
              n173 = while {
                shift-right: [w613] -> w605
                shift-left: w608 -> [w620]
                tunnel: w607 -> [w621]
                tunnel: [w611] -> w606
                stop <- w617 continue-if-true
                n174 = Preview Queue Element(queue=w621, timeout in ms (-1)=0, error in (no error)=w620) -> (element=w618:T7, timed out?=w615:bool, error out=w614:errorcluster)  [unwired: 1 out]
                n175 = global read "PauseMeander.vi" "Pause Meaner"() -> (w622:bool)
                n176 = Not Equal?(x=SequenceCtrl_State."Exit", y=w618) -> (x != y?=w616:bool)
                n177 = Compound Arithmetic op=AND(w616, invert w615) -> (w611:bool)
                n178 = Not(x=w611) -> (.not. x?=w610:bool)
                n179 = Or(x=w622, y=w611) -> (x .or. y?=w617:bool)
                n180 = call <userlib>:"Wait (ms)__ogtk.vi"("error in (no error)"=w614, "Wait on Error (FALSE)"=w610, "milliseconds to wait"=u32 200) -> ("error out"=w613:errorcluster)  [unwired: 7 in, 1 out]
              }
            }
            frame "Exit" {
              n181 = Enqueue Element At Opposite End(queue=w625, element=SequenceCtrl_State."Quit", error in (no error)=w641) -> (queue out=w637:refnum<queue>, error out=w638:errorcluster)  [unwired: 1 in, 1 out]
              n182 = Enqueue Element At Opposite End(queue=w637, element=SequenceCtrl_State."StopLaser", error in (no error)=w638) -> (queue out=w629:refnum<queue>, error out=w628:errorcluster)  [unwired: 1 in, 1 out]
              n183 = disable-structure shown="Enabled" {
                disable-tunnel: w629 -> [w645 _]
                disable-tunnel: w628 -> [w644 w647]
                disable-tunnel: [w643 w647] -> w627
                frame Disabled {
                  n184 = Enqueue Element At Opposite End(queue=w645, element=SequenceCtrl_State."EndOfLine", error in (no error)=w644) -> (error out=w643:errorcluster)  [unwired: 1 in, 2 out]
                }
                frame Enabled {
                }
              }
              n185 = Enqueue Element At Opposite End(queue=w640, element=T8 {"State"=enum."STOP", "Params."=variant}, error in (no error)=w627) -> ()  [unwired: 1 in, 3 out]
            }
            frame "RestoreVelocity" {
              # "handle leak"
              n186 = Enqueue Element(queue=w651, element=SequenceCtrl_State."CheckPause", error in (no error)=w652) -> (error out=w650:errorcluster)  [unwired: 1 in, 2 out]
              n187 = Obtain Queue(name (unnamed)="Motion_Status", element data type=T9 {"Position"=[], "Velocity"=[], "Acceleration"=[], "Moving"=FALSE, "Simulation"=FALSE, "tickcount_mov"=0, "tickcount_pos"=0, "NumOfAxis"=0, "Initialized"=FALSE, "CommPort"="", "Range"=[], "Serial Configuration"={"Baud Rate"=0, "Parity"=0, "Data Bits"=0, "Stop Bits"=0, "Flow Control"=0}, "MotorDisabled"=refnum}, error in (no error)=w650) -> (queue out=w665:refnum<queue>, error out=w664:errorcluster)  [unwired: 2 in, 1 out]
              n188 = Bundle By Name(cluster=T8 {"State"=enum."QueryStatus", "Params."=variant} ("element"), "Params."=w665) -> (w666:T8)
              n189 = Dequeue Element(queue=w665, error in (no error)=w664) -> (element=w663:T9, error out=w661:errorcluster)  [unwired: 1 in, 2 out]
              n190 = Enqueue Element(queue=w658, element=w666) -> (queue out=w669:refnum<queue>)  [unwired: 2 in, 2 out]
              n191 = Unbundle By Name(w663) -> ("NumOfAxis"=w662:i32)
              n192 = for {
                N: w662 -> [_]
                tunnel: w669 -> [w674]
                tunnel: w670 -> [w673]
                shift-right: [w671] -> w660
                shift-left: w661 -> [w672]
                i -> [w680]
                n193 = Increment(x=w680) -> (x+1=w678:i32)
                n194 = Bundle By Name(cluster=cluster{"Axis":i32, "Velocity":dbl} {"Axis"=0, "Velocity"=0.0}, "Velocity"=w673, "Axis"=w678) -> (w675:cluster{"Axis":i32, "Velocity":dbl})
                n195 = Bundle By Name(cluster=T8 {"State"=enum."SetVelocity", "Params."=variant} ("element"), "Params."=w675) -> (w677:T8)
                n196 = Enqueue Element(queue=w674, element=w677, error in (no error)=w672) -> (error out=w671:errorcluster)  [unwired: 1 in, 2 out]
              }
            }
            frame "Pause" {
              # "Not mature, skip"
              # "Stop stage, laser\nwait\nrestart stage, laser / Quit"
              n197 = while {
                shift-right: [w695] -> w692
                shift-left: w694 -> [w706]
                shift-right: [w697] -> w690
                shift-left: w691 -> [w707]
                stop <- w699 stop-if-true
                n198 = Preview Queue Element(queue=w707, timeout in ms (-1)=0, error in (no error)=w706) -> (queue out=w698:refnum<queue>, element=w704:T7, timed out?=w702:bool, error out=w701:errorcluster)
                n199 = call <userlib>:"Wait (ms)__ogtk.vi"("error in (no error)"=w701, "milliseconds to wait"=u32 200) -> ("error out"=w696:errorcluster)  [unwired: 8 in, 1 out]
                n200 = Equal?(x=T15."Pause", y=w704) -> (x = y?=w703:bool)
                n201 = Compound Arithmetic op=AND(w703, invert w702) -> (w699:bool)
                n202 = case shown="True" w699 {
                  tunnel: w698 -> [w710 w714]
                  tunnel: [w710 w713] -> w697
                  tunnel: w696 -> [w709 w712]
                  tunnel: [w709 w711] -> w695
                  frame False {
                  }
                  frame True {
                    n203 = Dequeue Element(queue=w714, error in (no error)=w712) -> (queue out=w713:refnum<queue>, error out=w711:errorcluster)  [unwired: 1 in, 2 out]
                  }
                }
              }
              n204 = One Button Dialog(message="Internal error. Unexpected pause frame.") -> ()  [unwired: 1 in, 1 out]
              n205 = Enqueue Element At Opposite End(queue=w690, element=SequenceCtrl_State."StartOfLine", error in (no error)=w692) -> (error out=w693:errorcluster)  [unwired: 1 in, 2 out]
            }
            frame "Quit" {
              w716 = TRUE
              # "Dupliate of \"restore high velocity\"\nOtherwise race condition may skip it"
              n206 = Obtain Queue(name (unnamed)="Status", element data type=T9 {"Position"=[], "Velocity"=[], "Acceleration"=[], "Moving"=FALSE, "Simulation"=FALSE, "tickcount_mov"=0, "tickcount_pos"=0, "NumOfAxis"=0, "Initialized"=FALSE, "CommPort"="", "Range"=[], "Serial Configuration"={"Baud Rate"=0, "Parity"=0, "Data Bits"=0, "Stop Bits"=0, "Flow Control"=0}, "MotorDisabled"=refnum}, error in (no error)=w717) -> (queue out=w730:refnum<queue>, error out=w729:errorcluster)  [unwired: 2 in, 1 out]
              n207 = Bundle By Name(cluster=T8 {"State"=enum."QueryStatus", "Params."=variant} ("element"), "Params."=w730) -> (w731:T8)
              n208 = Dequeue Element(queue=w730, error in (no error)=w729) -> (element=w728:T9, error out=w726:errorcluster)  [unwired: 1 in, 2 out]
              n209 = Enqueue Element(queue=w723, element=w731) -> (queue out=w734:refnum<queue>)  [unwired: 2 in, 2 out]
              n210 = Unbundle By Name(w728) -> ("NumOfAxis"=w727:i32)
              n211 = for {
                N: w727 -> [_]
                tunnel: w734 -> [w739]
                tunnel: w735 -> [w738]
                shift-right: [w736] -> w725
                shift-left: w726 -> [w737]
                i -> [w745]
                n212 = Increment(x=w745) -> (x+1=w743:i32)
                n213 = Bundle By Name(cluster=cluster{"Axis":i32, "Velocity":dbl} {"Axis"=0, "Velocity"=0.0}, "Velocity"=w738, "Axis"=w743) -> (w740:cluster{"Axis":i32, "Velocity":dbl})
                n214 = Bundle By Name(cluster=T8 {"State"=enum."SetVelocity", "Params."=variant} ("element"), "Params."=w740) -> (w742:T8)
                n215 = Enqueue Element(queue=w739, element=w742, error in (no error)=w737) -> (error out=w736:errorcluster)  [unwired: 1 in, 2 out]
              }
            }
          }
        }
        frame Error {
          n216 = Unbundle By Name(w753) -> ("source"=w752:string)
          n217 = Format Into String(w748) -> (resulting string=w749:string)  [unwired: 3 in, 1 out]
          n218 = Concatenate Strings(w752, w749) -> (w750:string)
          n219 = One Button Dialog(message=w750) -> ()  [unwired: 1 in, 1 out]
        }
      }
      n220 = call <userlib>:"ErrorLog.vi"("error in (no error)"=w97) -> ("error out"=w80:errorcluster)  [unwired: 10 in]
      "Core_iter." <- w84
    }
  }
  "Interupted" <- w42
  n221 = while {
    tunnel: "AppsRef" -> [w764]
    tunnel: w27 -> [w761]
    tunnel: "MotionStageRefs" -> [w760]
    shift-right: [w759] -> w21
    shift-left: FALSE -> [w758]
    stop <- w762 stop-if-true
    # "Interrupted Stop"
    n222 = Dequeue Element(queue=w764) -> (element=w763:T5)  [unwired: 2 in, 3 out]
    n223 = case shown="\"Interrupted_Stop\"" w763 {
      tunnel: [_ FALSE TRUE] -> w762
      tunnel: w761 -> [_ w773 _]
      tunnel: w760 -> [_ w770 _]
      tunnel: [w765 TRUE w775] -> w759
      tunnel: w758 -> [w765 _ w775]
      frame Default {
      }
      frame "Interrupted_Stop" {
        n224 = Enqueue Element At Opposite End(queue=w773, element=SequenceCtrl_State."Exit", timeout in ms (-1)=1000) -> (timed out?=→"timed out?":bool, error out=w768:errorcluster)  [unwired: 1 in, 1 out]
        n225 = Enqueue Element At Opposite End(queue=w770, element=T8 {"State"=enum."STOP", "Params."=variant}, error in (no error)=w768) -> ()  [unwired: 1 in, 3 out]
      }
      frame "Quit_SubProgram" {
      }
    }
  }
  n226 = Increment(x=w45) -> (x+1=→"Scanned Lines":i32)
  n227 = Unbundle By Name(w35) -> ("Feedback"=w34:refnum<queue>, "InfoRef"=w44:refnum<vi>)
  n228 = Release Queue "Only CoreLoop need it"(queue=w34, error in (no error)=w33) -> (error out=w32:errorcluster)  [unwired: 1 in, 2 out]
  n229 = property class="Str"(reference=w44, error in=w32, "Value"="") -> (error out=w36:errorcluster)  [unwired: 1 out]
  n230 = Release Queue(queue=w27, error in (no error)=w36) -> (error out=w24:errorcluster)  [unwired: 1 in, 2 out]
  n231 = Enqueue Element(queue="AppsRef", element=States-AToF."Quit_SubProgram", error in (no error)=w24) -> (error out=w22:errorcluster)  [unwired: 1 in, 2 out]
  n232 = case shown="True" w21 {
    tunnel: w22 -> [_ w777]
    tunnel: w14 -> [_ w780]
    frame False {
    }
    frame True {
      n233 = Generate User Event(user event=w780, event data cluster=cluster{"Quit":bool} {"Quit"=TRUE} ("event data"), error in=w777) -> (error out=w778:errorcluster)  [unwired: 1 in, 1 out]
      n234 = call <vilib>:"Clear Errors.vi"("error in (no error)"=w778) -> ()  [unwired: 5 in, 2 out]
    }
  }
  n235 = Enqueue Element At Opposite End(queue="AppsRef", element=States-AToF."Interrupted_Stop", timeout in ms (-1)=1000, error in (no error)=w12) -> (error out=w31:errorcluster)  [unwired: 2 out]
  n236 = call <vilib>:"Clear Errors.vi"("error in (no error)"=w31) -> ("error out"=w25:errorcluster)  [unwired: 5 in, 1 out]
  n237 = Merge Errors(w25, w22) -> (w23:errorcluster)
  n238 = Release Queue(queue=w20, error in (no error)=w23) -> (error out=→"error out":errorcluster)  [unwired: 1 in, 2 out]
